vi "KM_control.vi"() -> ()   [LabVIEW 2015]
uses:
  <instrlib>/Zurich Instruments LabOne/Zurich Instruments LabOne.lvlib
panel:
  in  "Abort":bool
  in  "stop":bool
  out "Selected Device":string
  in  "Address":string="DEV"
  in  "Log Sweep":bool
  in  "Averaging":u16(ring)=1 items=["1"=1, "2"=2, "4"=4, "16"=16, "32"=32, "64"=64]
  in  "Bandwidth (Hz)":dbl=-1.0 format="%#_p"
  in  "Precision":u16(ring) items=["Low", "Med", "High"]
  in  "Number of Points":i32=100 caption="Points" min=2 max=66000
  in  "Filter Order":i32(ring)=4 items=["6, 1st"=1, "12, 2nd"=2, "18, 3rd"=3, "24, 4th"=4, "30, 5th"=5, "36, 6th"=6, "42, 7th"=7, "48, 8th"=8]
  in  "Stop (Hz)":dbl=1000000.0 format="%_5p"
  in  "Start (Hz)":dbl=10000.0 format="%_5p"
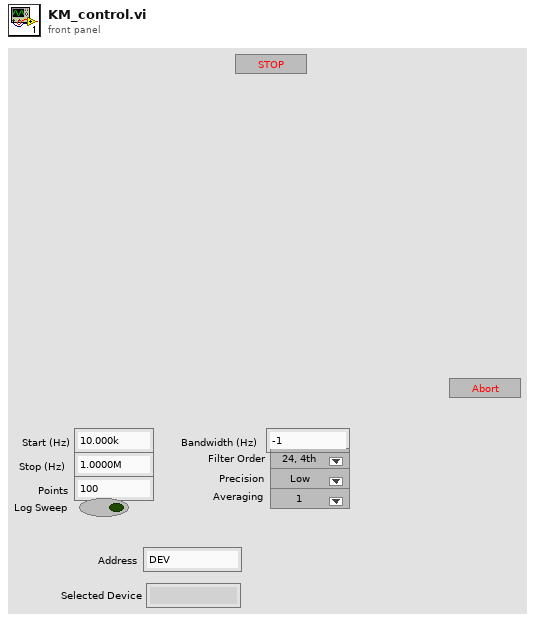
[diagram p1: front panel]
types:
  T1 = typedef "Zurich Instruments LabOne.lvlib/ziTypeHandle.ctl" = cluster{"handleValid":bool, "Conn":u64, "Path Prefix":string, "Handle":u64, "Connected":bool, "Clockbase(s)":dbl}
  T2 = cluster{"Output (F,X1,Y1,X2,Y2,...,Vo)":dbl[][], "Point (#)":i32}
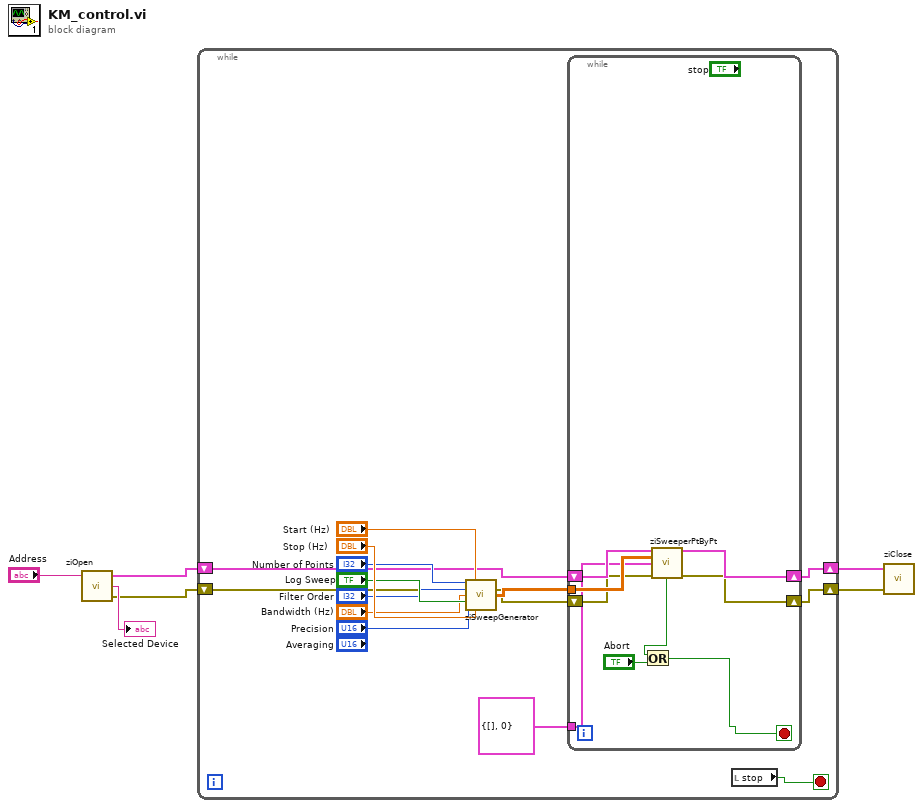
[diagram p0: block diagram]
diagram:
  n1 = call <instrlib>:"ziOpen.vi"("Address"="Address") -> ("Error Out"=w3:errorcluster, "Selected Device"=→"Selected Device":string, "HandleOut"=w4:T1)  [unwired: 3 in]
  n2 = while {
    shift-right: [w9] -> w2
    shift-left: w4 -> [w12]
    shift-right: [w8] -> w1
    shift-left: w3 -> [w11]
    stop <- w7 stop-if-true
    n3 = call <instrlib>:"ziSweepGenerator.vi"("Steps (#)"="Number of Points", "Start (Hz)"="Start (Hz)", "Order (4)"="Filter Order", "Bandwith (-1=auto)"="Bandwidth (Hz)", "Log Sweep (true)"="Log Sweep", "Precision (Low)"="Precision", "Stop (Hz)"="Stop (Hz)") -> ("Sweep Sequence (F (Hz), BW (Hz), TC(s), Time(s))"=w13:dbl[][])  [unwired: 6 in, 2 out]
    n4 = while {
      tunnel: w13 -> [w29]
      tunnel: T2 {"Output (F,X1,Y1,X2,Y2,...,Vo)"=[], "Point (#)"=0} ("State Out") -> [w26]
      shift-right: [w25] -> w9
      shift-left: w12 -> [w28]
      shift-right: [w24] -> w8
      shift-left: w11 -> [w27]
      stop <- w21 stop-if-true
      n5 = call <instrlib>:"ziSweeperPtByPt.vi"("Handle In"=w28, "Sweep Sequence In"=w29, "State In"=w26, "Error In"=w27) -> ("Handle Out"=w25:T1, "Done"=w22:bool, "Error Out"=w24:errorcluster)  [unwired: 8 in, 1 out]
      n6 = Or(x=w22, y="Abort") -> (x .or. y?=w21:bool)
    }
    n7 = local read "stop"() -> (w7:bool)
  }
  n8 = call "ziClose.vi"("Error In"=w1, "Handle In"=w2) -> ()  [unwired: 2 in, 2 out]
